vi "XIPIN_Clocking_Wizard_3_6.vi"   [LabVIEW 2017]
doc: "This is Rev3 version of Clocking Wizard v3.6. The Clocking Wizard creates an HDL file (Verilog or VHDL) that contains a clocking circuit customized to the user's clocking requirements.\n------------------------------------\n<b>Need License</b> : No"
uses:
  <vilib>/rvi/XilinxIP/XIPIN_XNode/niFpgaXIPIN.xnode
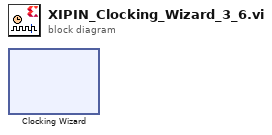
[diagram p0: block diagram]
diagram:
  n1 = xnode ("Clocking Wizard")() -> ()
